vi "Close.vi"(8 "error in (no error)":errorcluster, 11 "AudioOut (N Samples) Ref In":T1) -> (0 "error out":errorcluster)   [LabVIEW 2021, in "AudioOut Block.lvlib"]
doc: "Closes the reference to one or more audio output channels, which you use to perform n samples write operations."
uses:
  <vilib>/myRIO/Instrument Drivers/Onboard IO/AudioOut Block/AudioOut Block.lvlib
  <vilib>/myRIO/Instrument Drivers/Onboard IO/AudioOut Block/typedefs/AudioOut Block Reference.ctl
  <vilib>/myRIO/Common/Instrument Driver Framework/Utilities/typedefs/myRIO Generic Hardware Reference.ctl
  <vilib>/myRIO/Common/Instrument Driver Framework/Utilities/typedefs/Hardware Version Enum.ctl
  <vilib>/myRIO/Common/Instrument Driver Framework/Utilities/typedefs/myRIO v1.0 Reference.ctl
  <vilib>/myRIO/Common/Instrument Driver Framework/Utilities/typedefs/Generic FPGA Reference.ctl
  <vilib>/myRIO/Common/Instrument Driver Framework/myRIO v1.0/AudioOut Block/typedefs/AudioOut Block Channels List.ctl
  <vilib>/myRIO/Common/Instrument Driver Framework/myRIO v1.0/AudioOut Block/typedefs/AudioOut Block Channels Enum.ctl
  <vilib>/myRIO/Common/Instrument Driver Framework/Utilities/typedefs/Analog Scaling Constants.ctl
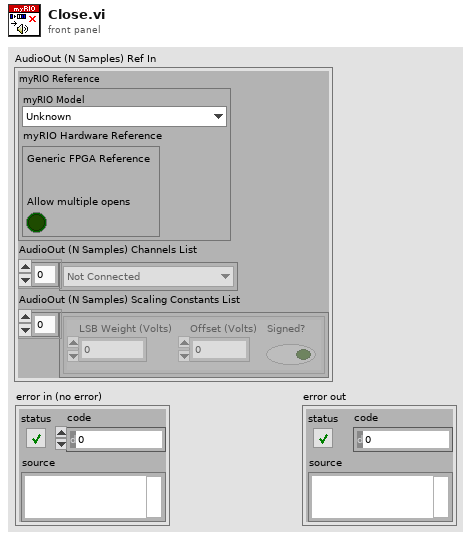
[diagram p1: front panel]
types:
  T1 = typedef "AudioOut Block.lvlib/AudioOut Block Reference.ctl" = cluster{"myRIO Reference":T2, "AudioOut (N Samples) Channels List":T6, "AudioOut (N Samples) Scaling Constants List":T8[]}
  T2 = typedef "myRIO Generic Hardware Reference.ctl" = cluster{"myRIO Model":T3, "myRIO Hardware Reference":T4}
  T3 = typedef "Hardware Version Enum.ctl" = enum16{"Unknown", "myRIO-1900", "myRIO-1950", "roboRIO", "NI ELVIS RIO CM", "ELVIS III"}
  T4 = typedef "myRIO v1.0 Reference.ctl" = cluster{"Generic FPGA Reference":T5, "Allow multiple opens":bool}
  T5 = typedef "Generic FPGA Reference.ctl" = refnum<k20>
  T6 = typedef "AudioOut Block Channels List.ctl" = T7[]
  T7 = typedef "AudioOut Block Channels Enum.ctl" = enum16{"Not Connected", "AudioOut/Left (N Samples)", "AudioOut/Right (N Samples)"}
  T8 = typedef "Analog Scaling Constants.ctl" = cluster{"LSB Weight (Volts)":dbl, "Offset (Volts)":dbl, "Signed?":bool}
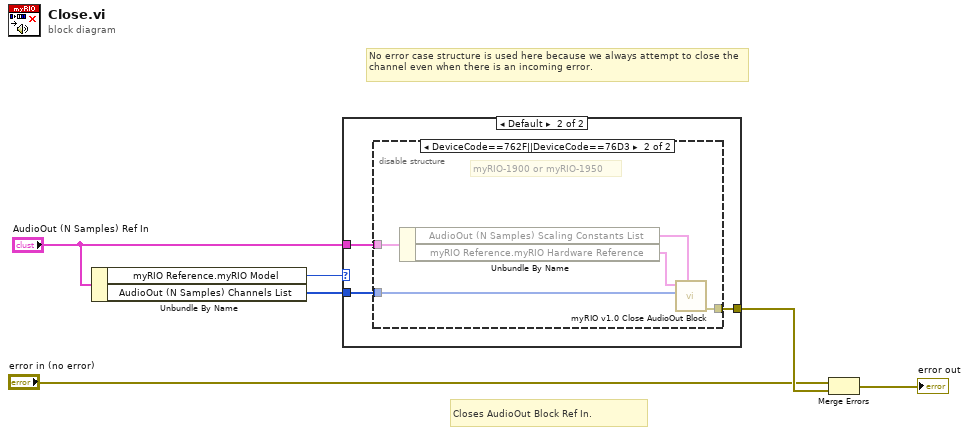
[diagram p0: block diagram]
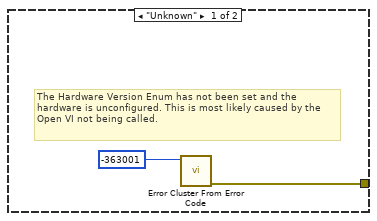
[diagram p2: hidden frame]
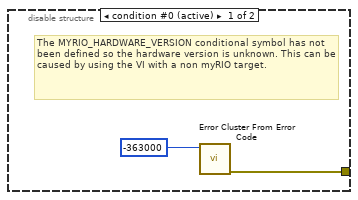
[diagram p3: hidden frame]
diagram:
  # "No error case structure is used here because we always attempt to close the channel even when there is an incoming error."
  # "Closes AudioOut Block Ref In."
  n1 = Unbundle By Name("AudioOut (N Samples) Ref In") -> ("myRIO Reference.myRIO Model"=w5:T3, "AudioOut (N Samples) Channels List"=w6:T6)
  n2 = case shown="Default" w5 {
    tunnel: "AudioOut (N Samples) Ref In" -> [_ w11]
    tunnel: [w7 w10] -> w4
    tunnel: w6 -> [_ w9]
    frame "Unknown" {
      # "The Hardware Version Enum has not been set and the hardware is unconfigured. This is most likely caused by the Open VI not being called."
      n3 = call <vilib>:"Error Cluster From Error Code.vi"("error code (0)"=-363001) -> ("error out"=w7:errorcluster)  [unwired: 8 in]
    }
    frame Default {
      n4 = disable-structure shown="DeviceCode==762F||DeviceCode==76D3" {
        disable-tunnel: w11 -> [_ w18]
        disable-tunnel: [w12 w17] -> w10
        disable-tunnel: w9 -> [_ w16]
        frame condition #0 (active) {
          # "The MYRIO_HARDWARE_VERSION conditional symbol has not been defined so the hardware version is unknown. This can be caused by using the VI with a non myRIO target."
          n5 = call <vilib>:"Error Cluster From Error Code.vi"("error code (0)"=-363000) -> ("error out"=w12:errorcluster)  [unwired: 8 in]
        }
        frame condition #1 {
          # "myRIO-1900 or myRIO-1950"
          n6 = Unbundle By Name(w18) -> ("AudioOut (N Samples) Scaling Constants List"=w14:T8[], "myRIO Reference.myRIO Hardware Reference"=w15:T4)
          n7 = call <vilib>:"myRIO v1.0 Close AudioOut Block.vi"("Scaling Constants List"=w14, "AudioOut (N Samples) Channel List"=w16, "myRIO Ref In"=w15) -> ("error out"=w17:errorcluster)  [unwired: 8 in]
        }
      }
    }
  }
  n8 = Merge Errors("error in (no error)", w4) -> (→"error out":errorcluster)
